vi "Process.vi"(11 "Test Actor":refnum<class "Test Actor.lvclass">) -> ()   [LabVIEW 2020, in "Test Actor.lvclass"]
uses:
  Test Actor.lvclass
  C:/Users/neilp/Desktop/Actors/Actor/Actor/Actor.lvclass
  Test Actor.lvclass/Test Actor.ctl
  Count Behaviour.ctl
  Base Actor/Actor/Actor.lvclass
panel:
  out "Numeric":i32
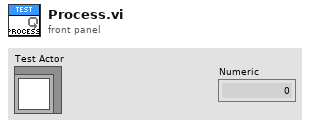
[diagram p1: front panel]
types:
  T1 = typedef "Test Actor.lvclass/Count Behaviour.ctl" = enum16{"Stopped", "Up", "Down"}
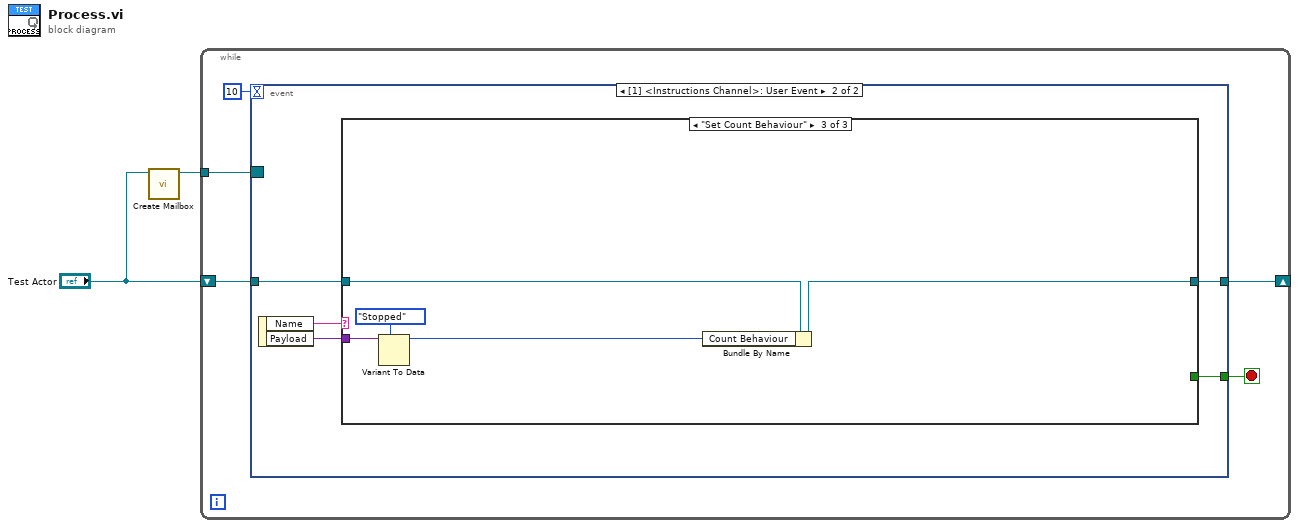
[diagram p0: block diagram]
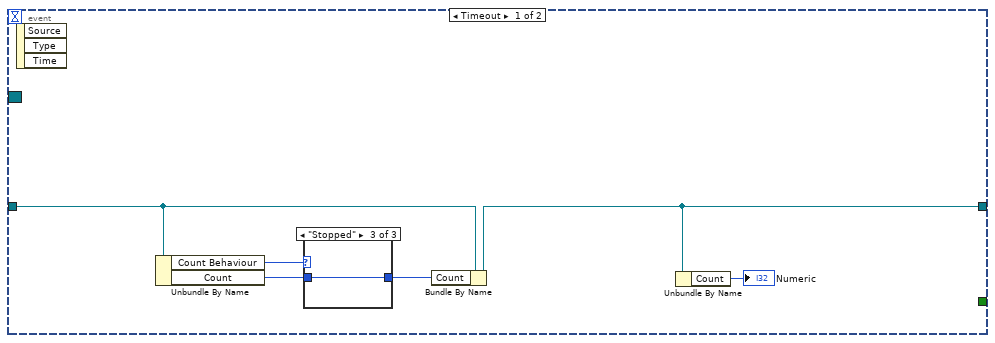
[diagram p2: hidden frame]
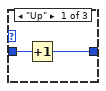
[diagram p3: hidden frame]
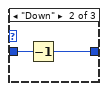
[diagram p4: hidden frame]
diagram:
  n1 = call "Create Mailbox.vi"("Actor in"="Test Actor") -> ("Mailbox"=w1:refnum<event-registration>)  [unwired: 9 in, 1 out]
  n2 = while {
    tunnel: w1 -> [w7]
    shift-right: [w3] -> _
    shift-left: "Test Actor" -> [w4]
    stop <- w6 stop-if-true
    n3 = event shown="[1] <Instructions Channel>: User Event" {
      selector: w7 -> [_ _]
      dyn-events: _ -> [_ _]
      timeout: 10 -> [_ _]
      tunnel: [_ w21] -> w6
      tunnel: w4 -> [w12 w20]
      tunnel: [w10 w19] -> w3
      event Timeout {
        n4 = event-data() -> ()  [unwired: 1 in, 3 out]
        n5 = Unbundle By Name(w12) -> ("Count Behaviour"=w8:T1, "Count"=w13:i32)
        n6 = case shown="\"Stopped\"" w8 {
          tunnel: w13 -> [w15 w17 w18]
          tunnel: [w14 w16 w18] -> w11
          frame "Up" {
            n7 = Increment(x=w15) -> (x+1=w14:i32)
          }
          frame "Down" {
            n8 = Decrement(x=w17) -> (x-1=w16:i32)
          }
          frame "Stopped" {
          }
        }
        n9 = Bundle By Name(cluster=w12, "Count"=w11) -> (w10:refnum<class "Test Actor.lvclass">)
        n10 = Unbundle By Name(w10) -> ("Count"=→"Numeric":i32)
      }
      event User Event {
        n11 = event-data() -> ("Name"=w23:string, "Payload"=w22:variant)  [unwired: 1 in]
        n12 = case shown="\"Set Count Behaviour\"" w23 {
          tunnel: w22 -> [_ _ w29]
          tunnel: [_ TRUE _] -> w21
          tunnel: w20 -> [w24 w25 w30]
          tunnel: [w24 w25 w31] -> w19
          frame Default {
          }
          frame "Shutdown" {
          }
          frame "Set Count Behaviour" {
            n13 = Variant To Data(type=Count_Behaviour."Stopped" ("Count Behaviour"), Variant=w29) -> (data=w27:T1)  [unwired: 1 in, 1 out]
            n14 = Bundle By Name(cluster=w30, "Count Behaviour"=w27) -> (w31:refnum<class "Test Actor.lvclass">)
          }
        }
      }
    }
  }
